vi "_Remote RT Copy.vi"(6 "Error In":errorcluster, 7 "Copy software only":bool, 8 "Image Destination":T1, 9 "Image Source":T1) -> (0 "Error Out":errorcluster, 3 "Messages":string)   [LabVIEW 2018]
uses:
  Type/_RT Command.ctl
  Type/_RT Instrument State.ctl
  Configuration/_Global Configuration.vi
  <vilib>/nisyscfg/Create System Image (Folder).vi
  <vilib>/nisyscfg/Set System Image (Folder).vi
  <vilib>/nisyscfg/Close (System).vi
  <vilib>/nisyscfg/nisyscfg.lvlib
panel:
  out "IP Address:":string
  out "Current Task":string
  # "Please wait up to a few minutes while copying firmware"
  # "(This dialog will automatically close when update is finished)"
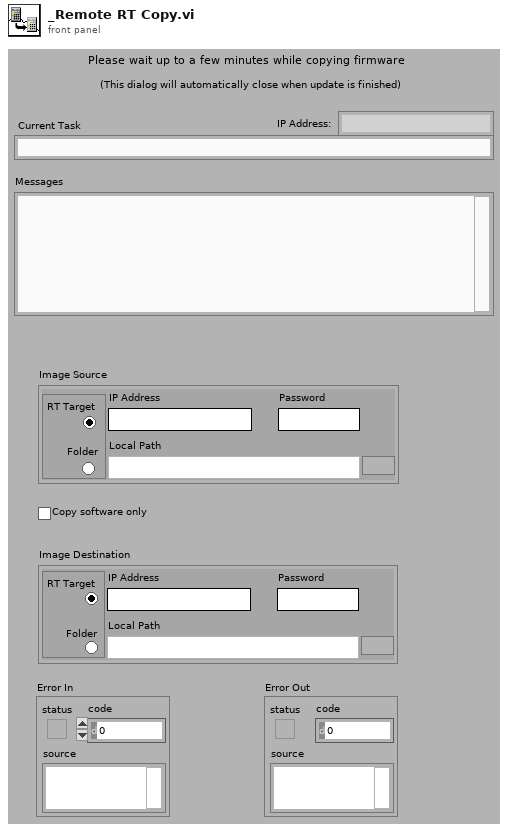
[diagram p1: front panel]
types:
  T1 = cluster{"IP Address":string, "Password ":string, "Local Path":path, "Radio Buttons":enum32{"RT Target", "Folder"}}
  T2 = typedef "_RT Command.ctl" = enum16{"xml Start Run", "xml Start Actual Run", "xml Stop Run", "xml Runtime Update", "xml Get Status", "xml Get Table", "xml Set Table", "xml Get Configuration", "xml System Status", "xml Set LC Input Logic", "xml Get Data", "xml Get Info", "Start", "StartActualRun", "Stop", "Runtime Update", "Get Data", "Get Info", "Get Status", "Get Param", "Get Config", "Get Table", "Read ADC", "Set Oscillator", "Update Config", "Update Table", "Set All Pol", "Set Pol and DC", "Set Max Mass", "Toggle RP", "Toggle EL", "Set PIC", "Initialize Turbo", "Send Turbo Comm", "Close Turbo", "P1", "P2", "P3", "Send Serial", "Set LC Out", "Get LC In", "Read VAC", "Test Table", "Toggle Power", "Get Startup", "Set Startup", "Get ADC Table", "Set ADC Table", "Get Brief Status", "Get Detail Status", "Auxiliary Update", "Set CC Logics", "Set CC Input Logics", "Ignore Error", "invalid"}
  T3 = enum16{"Use Dialog", "Temporary File", "My Tables"}
  T4 = typedef "_RT Instrument State.ctl" = enum16{"Initializing", "Mass Spectrometer is Off", "Starting Up", "Turning Power Off", "Going to Standby", "Roughing Pump Ready", "Turning Turbo Off", "Turbo Startup", "Turbopump Ready", "Checking Vacuum", "Going to Ready", "Ready", "Running", "Source Standby", "Lost Communication", "Shutting Down", "Fault", "24V Standby", "Go to 24V Standby", "Turbopump Ready-Waiting"}
  T5 = cluster{"Model":string, "MAC Address":string, "Hostname":string}
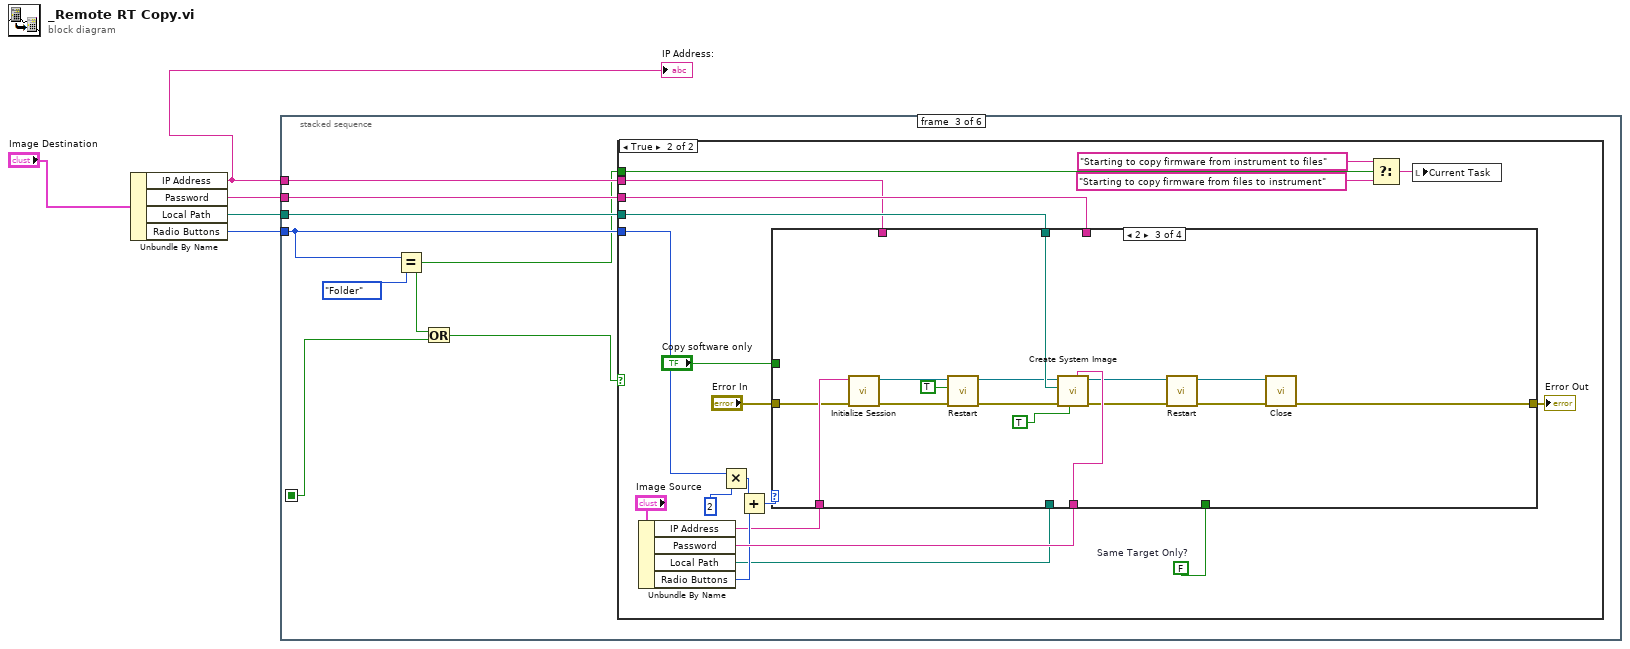
[diagram p0: block diagram]
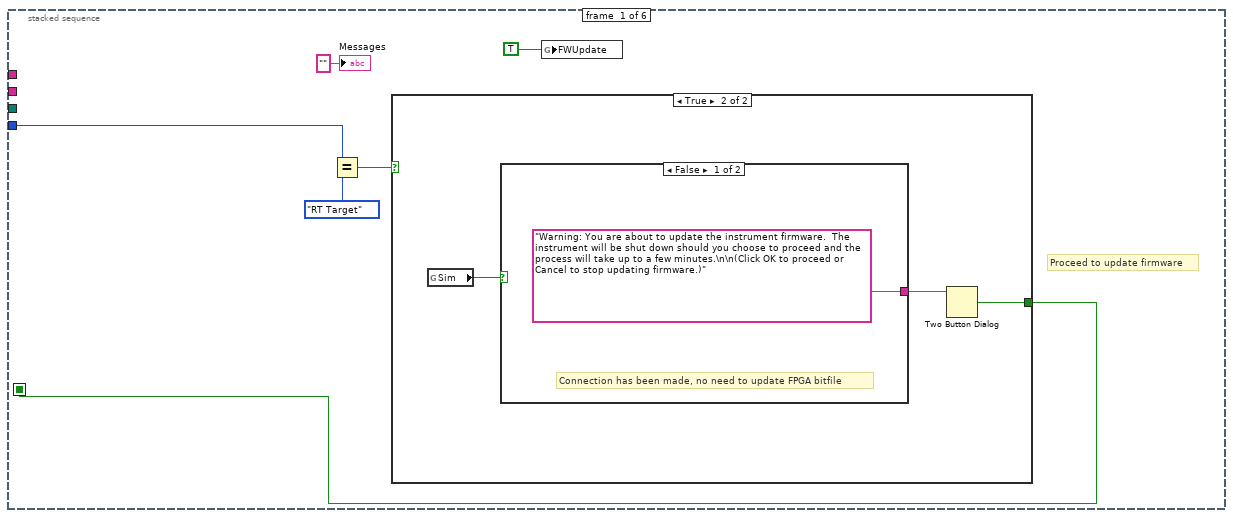
[diagram p2: hidden frame]
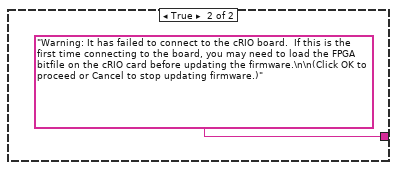
[diagram p4: hidden frame]
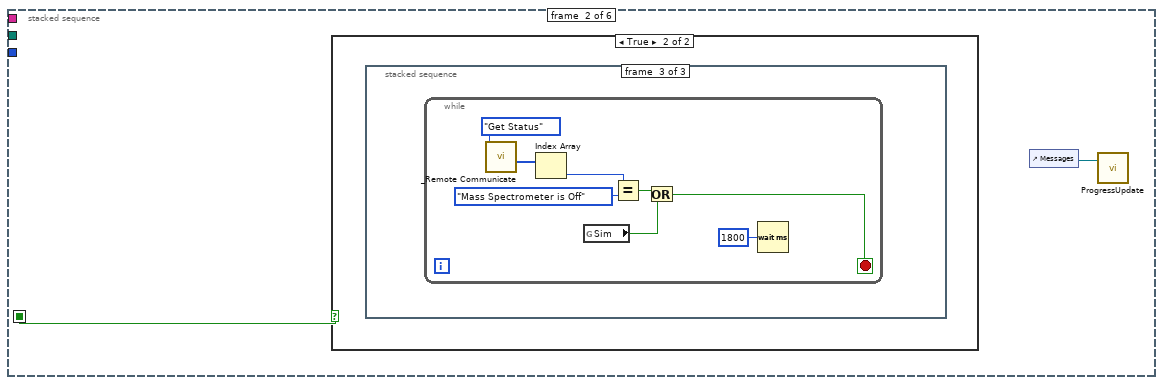
[diagram p5: hidden frame]
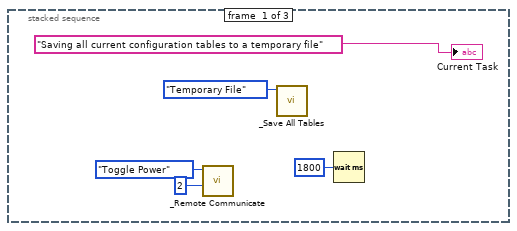
[diagram p7: hidden frame]
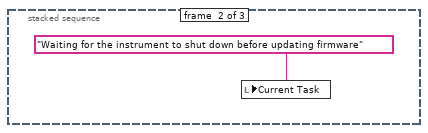
[diagram p8: hidden frame]
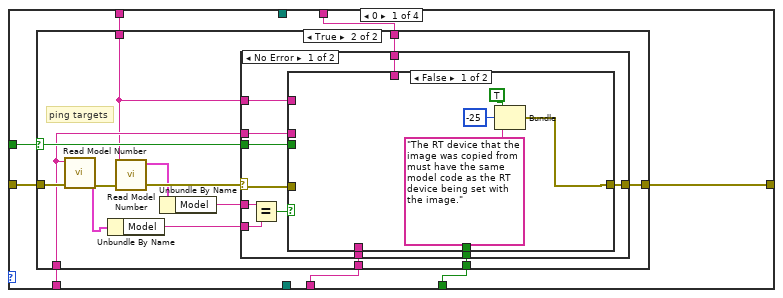
[diagram p10: hidden frame]
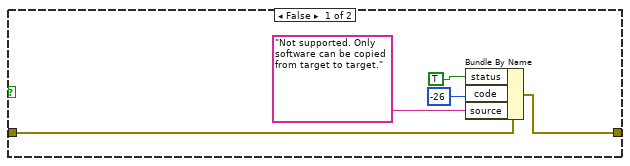
[diagram p11: hidden frame]
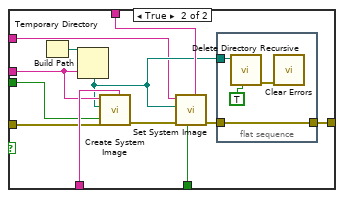
[diagram p12: hidden frame]
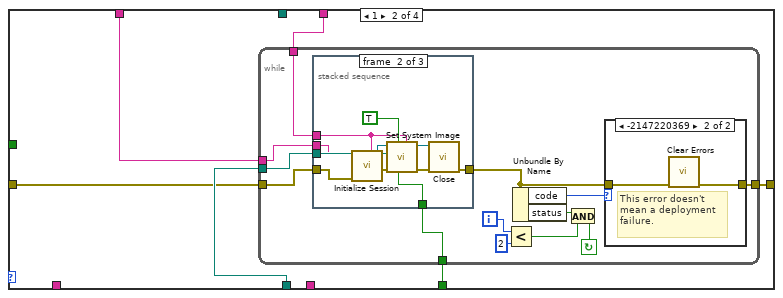
[diagram p14: hidden frame]
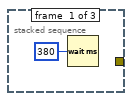
[diagram p16: hidden frame]
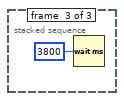
[diagram p17: hidden frame]
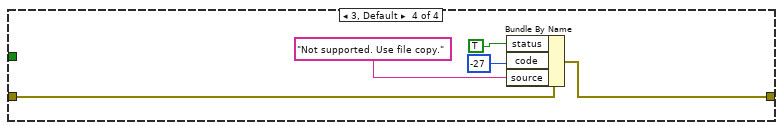
[diagram p18: hidden frame]
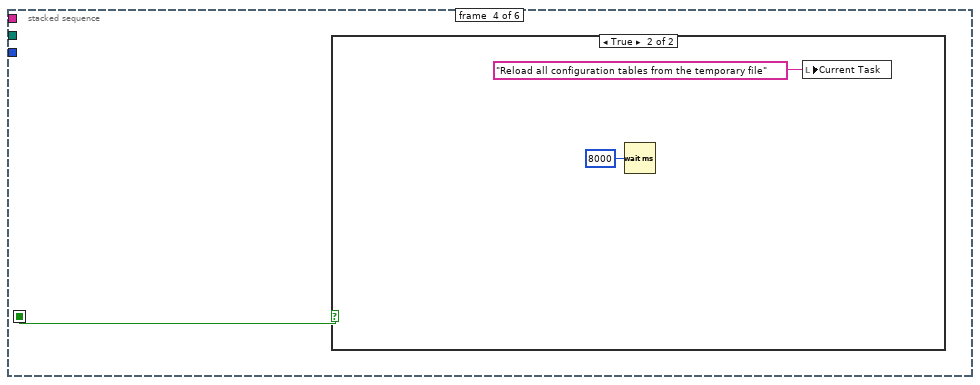
[diagram p19: hidden frame]
diagram:
  n1 = Unbundle By Name("Image Destination") -> ("IP Address"=w1:string, "Password"=w4:string, "Local Path"=w3:path, "Radio Buttons"=w2:enum32{"RT Target", "Folder"})
  "IP Address:" <- w1
  n2 = stacked-sequence {
    seq-local: [w8 _ _ _ _ _] -> [_ w19 w35 w176 w180 _]
    tunnel: w2 -> [w10 _ w37 _ _ _]
    tunnel: w4 -> [_ _ w41 _ _ _]
    tunnel: w3 -> [_ _ w40 _ _ _]
    tunnel: w1 -> [_ _ w39 _ w179 _]
    frame #0 {
      # "Proceed to update firmware"
      n3 = Equal?(x=w10, y=enum32{"RT Target", "Folder"}."RT Target") -> (x = y?=w9:bool)
      n4 = case shown="True" w9 {
        selector: w9 -> [w12 _]
        tunnel: [w12 w15] -> w8
        frame False {
        }
        frame True {
          n5 = global read "_Global Configuration.vi" "Sim"() -> (w13:bool)
          n6 = case shown="False" w13 {
            tunnel: ["Warning: You are about to update the instrument firmware.  The instrument will be shut down should you choose to proceed and the process will take up to a few minutes.\n\n(Click OK to proceed or Cancel to stop updating firmware.)" "Warning: It has failed to connect to the cRIO board.  If this is the first time connecting to the board, you may need to load the FPGA bitfile on the cRIO card before updating the firmware.\n\n(Click OK to proceed or Cancel to stop updating firmware.)"] -> w14
            frame False {
              # "Connection has been made, no need to update FPGA bitfile"
            }
            frame True {
            }
          }
          n7 = Two Button Dialog(message=w14) -> (T button?=w15:bool)  [unwired: 2 out]
        }
      }
      n8 = global write "_Global Configuration.vi" "FWUpdate"(TRUE ("Update")) -> ()
      "Messages" <- "" ("Messages")
    }
    frame #1 {
      n9 = case shown="True" w19 {
        frame False {
        }
        frame True {
          n10 = stacked-sequence {
            frame #0 {
              n11 = call "_Remote Communicate.vi"("DC Param"=u16 2, "Command"=_RT_Command."Toggle Power") -> ()  [unwired: 4 in, 4 out]
              n12 = call "_Save All Tables.vi"("SaveOption (Temporary File)"=T3."Temporary File" ("Use temporary file (F)")) -> ()  [unwired: 2 in, 5 out]
              n13 = Wait (ms)(milliseconds to wait=u32 1800) -> ()  [unwired: 1 out]
              "Current Task" <- "Saving all current configuration tables to a temporary file"
            }
            frame #1 {
              n14 = local write "Current Task"("Waiting for the instrument to shut down before updating firmware") -> ()
            }
            frame #2 {
              n15 = while {
                stop <- w27 stop-if-true
                n16 = call "_Remote Communicate.vi"("Command"=_RT_Command."Get Status") -> ("Data Array"=w32:i32[])  [unwired: 5 in, 3 out]
                n17 = Index Array(array=w32) -> (element=w31:i32)  [unwired: 1 in]
                n18 = global read "_Global Configuration.vi" "Sim"() -> (w28:bool)
                n19 = Equal?(x=w31, y=_RT_Instrument_State."Mass Spectrometer is Off" ("InstrState")) -> (x = y?=w29:bool)
                n20 = Or(x=w29, y=w28) -> (x .or. y?=w27:bool)
                n21 = Wait (ms)(milliseconds to wait=u32 1800) -> ()  [unwired: 1 out]
              }
            }
          }
        }
      }
      n22 = control-ref of="Messages"() -> (w18:refnum<vi>)
      n23 = call <userlib>:"ProgressUpdate.vi"("Progress ref"=w18) -> ()  [unwired: 1 in, 1 out]
    }
    frame #2 {
      n24 = Equal?(x=w37, y=enum32{"RT Target", "Folder"}."Folder") -> (x = y?=w34:bool)
      n25 = Or(x=w34, y=w35) -> (x .or. y?=w36:bool)
      n26 = case shown="True" w36 {
        tunnel: w37 -> [_ w58]
        tunnel: w41 -> [_ w56]
        tunnel: w40 -> [_ w51]
        tunnel: w39 -> [_ w47]
        tunnel: w34 -> [_ w42]
        frame False {
        }
        frame True {
          w46 = FALSE  # Same Target Only?
          n27 = Unbundle By Name("Image Source") -> ("IP Address"=w48:string, "Password"=w55:string, "Local Path"=w52:path, "Radio Buttons"=w53:enum32{"RT Target", "Folder"})
          n28 = Multiply(x=w58, y=2) -> (x*y=w54:u32)
          n29 = Add(x=w54, y=w53) -> (x+y=w60:u32)
          n30 = case shown="2" w60 {
            tunnel: w47 -> [w68 w126 _ _]
            tunnel: w56 -> [w69 w122 _ _]
            tunnel: w48 -> [w66 _ w167 _]
            tunnel: w55 -> [w67 _ w165 _]
            tunnel: "Copy software only" -> [w63 _ _ _]
            tunnel: w52 -> [_ w125 _ _]
            tunnel: w51 -> [_ _ w170 _]
            tunnel: "Error In" -> [w64 w123 w166 w172]
            tunnel: [w65 w124 w168 w171] -> w49
            tunnel: w46 -> [w62 w121 _ _]
            frame 0 {
              n31 = case shown="True" w63 {
                selector: w63 -> [_ w87]
                tunnel: w69 -> [_ w86]
                tunnel: w68 -> [_ w81]
                tunnel: w67 -> [_ w88]
                tunnel: w66 -> [_ w82]
                tunnel: [w71 w85] -> w65
                tunnel: w64 -> [w72 w83]
                tunnel: w62 -> [_ w79]
                frame False {
                  n32 = Bundle By Name(cluster=w72, "status"=TRUE, "code"=-26, "source"="Not supported. Only software can be copied from target to target.") -> (w71:errorcluster)
                }
                frame True {
                  # "ping targets"
                  n33 = call "Read Model Number.vi"("error in (no error)"=w83, "String"=w82) -> ("error out"=w84:errorcluster, "Target Info"=w76:T5)  [unwired: 8 in]
                  n34 = Unbundle By Name(w76) -> ("Model"=w77:string)
                  n35 = call "Read Model Number.vi"("error in (no error)"=w84, "String"=w81) -> ("error out"=w80:errorcluster, "Target Info"=w75:T5)  [unwired: 8 in]
                  n36 = Unbundle By Name(w75) -> ("Model"=w78:string)
                  n37 = case shown="No Error" w80 {
                    selector: w80 -> [w95 w120]
                    tunnel: w88 -> [w99 _]
                    tunnel: w87 -> [w98 _]
                    tunnel: w86 -> [w92 _]
                    tunnel: [w97 w120] -> w85
                    tunnel: w82 -> [w94 _]
                    tunnel: w81 -> [w96 _]
                    tunnel: w79 -> [w93 _]
                    tunnel: w78 -> [w89 _]
                    tunnel: w77 -> [w91 _]
                    frame No Error {
                      n38 = Equal?(x=w89, y=w91) -> (x = y?=w90:bool)
                      n39 = case shown="False" w90 {
                        tunnel: w99 -> [_ w114]
                        tunnel: w98 -> [_ w113]
                        tunnel: [w100 w110] -> w97
                        tunnel: w96 -> [_ w104]
                        tunnel: w95 -> [_ w109]
                        tunnel: w94 -> [_ w106]
                        tunnel: w93 -> [_ w108]
                        tunnel: w92 -> [_ w107]
                        frame False {
                          n40 = Bundle("status"=TRUE, "code"=-25, "source"="The RT device that the image was copied from must have the same model code as the RT device being set with the image.") -> (w100:errorcluster)  [unwired: 1 out]
                        }
                        frame True {
                          n41 = Temporary Directory() -> (w115:path)
                          n42 = Build Path(base path=w115, name or relative path=w106) -> (appended path=w105:path)
                          n43 = call-poly <vilib>:"Create System Image.vi"("Encryption Passphrase"=w114, "Overwrite (F)"=w113, "error in (no error)"=w109, "Destination Folder"=w105, "Session in"=w106) -> ("error out"=w112:errorcluster)  [unwired: 4 in, 2 out]
                          n44 = call-poly <vilib>:"Set System Image.vi"("Encryption Passphrase"=w107, "Original System Only (F)"=w108, "error in (no error)"=w112, "Source Folder"=w105, "Session in"=w104) -> ("error out"=w111:errorcluster)  [unwired: 5 in, 1 out]
                          n45 = flat-sequence {
                            tunnel: w111 -> [w119]
                            tunnel: [w119] -> w110
                            tunnel: w105 -> [w117]
                            frame #0 {
                              n46 = call <vilib>:"Delete Directory Recursive.vi"("keep deleting on error? (F)"=TRUE, "Folder to Delete"=w117) -> ("error out"=w116:errorcluster)  [unwired: 1 in, 8 out]
                              n47 = call <vilib>:"Clear Errors.vi"("error in (no error)"=w116) -> ()  [unwired: 1 in, 6 out]
                            }
                          }
                        }
                      }
                    }
                    frame Error {
                    }
                  }
                }
              }
            }
            frame 1 {
              n48 = while {
                tunnel: w126 -> [w139]
                tunnel: w125 -> [w138]
                tunnel: [w128] -> w124
                tunnel: w123 -> [w137]
                tunnel: w122 -> [w136]
                tunnel: w121 -> [w135]
                i -> [w132]
                stop <- w134 continue-if-true
                n49 = stacked-sequence {
                  tunnel: w139 -> [_ w145 _]
                  tunnel: w138 -> [_ w154 _]
                  tunnel: w137 -> [_ w148 _]
                  tunnel: w136 -> [_ w146 _]
                  tunnel: w135 -> [_ w153 _]
                  tunnel: [_ w149 _] -> w129
                  frame #0 {
                    n50 = Wait (ms)(milliseconds to wait=u32 380) -> ()  [unwired: 1 out]
                  }
                  frame #1 {
                    n51 = call <vilib>:"Initialize Session.vi"("Password"=w146, "error in (no error)"=w148, "Target (localhost)"=w145) -> ("error out"=w147:errorcluster, "Session out"=w144:refnum<k21>)  [unwired: 7 in]
                    n52 = call-poly <vilib>:"Set System Image.vi"("Encryption Passphrase"=w146, "Original System Only (F)"=w153, "Restart Automatically (T)"=TRUE, "error in (no error)"=w147, "Source Folder"=w154, "Session in"=w144) -> ("error out"=w150:errorcluster, "Session out"=w151:refnum<k21>)  [unwired: 4 in]
                    n53 = call-poly <vilib>:"Close.vi"("error in (no error)"=w150, "Session in"=w151) -> ("error out"=w149:errorcluster)  [unwired: 9 in]
                  }
                  frame #2 {
                    n54 = Wait (ms)(milliseconds to wait=u32 3800) -> ()  [unwired: 1 out]
                  }
                }
                n55 = Less?(x=w132, y=2) -> (x < y?=w130:bool)
                n56 = Unbundle By Name(w129) -> ("code"=w127:i32, "status"=w133:bool)
                n57 = And(x=w133, y=w130) -> (x .and. y?=w134:bool)
                n58 = case shown="-2147220369" w127 {
                  tunnel: w129 -> [w140 w142]
                  tunnel: [w140 w141] -> w128
                  frame Default {
                  }
                  frame -2147220369 {
                    # "This error doesn't\nmean a deployment\nfailure."
                    n59 = call <vilib>:"Clear Errors.vi"("error in (no error)"=w142) -> ("error out"=w141:errorcluster)  [unwired: 5 in, 1 out]
                  }
                }
              }
            }
            frame 2 {
              n60 = call <vilib>:"Initialize Session.vi"("error in (no error)"=w166, "Target (localhost)"=w167) -> ("error out"=w162:errorcluster, "Session out"=w164:refnum<k21>)  [unwired: 8 in]
              n61 = call <vilib>:"Restart.vi"("error in (no error)"=w162, "Install Mode (F)"=TRUE, "Session in"=w164) -> ("error out"=w161:errorcluster, "Session out"=w163:refnum<k21>)  [unwired: 6 in, 1 out]
              n62 = call-poly <vilib>:"Create System Image.vi"("Encryption Passphrase"=w165, "Overwrite (F)"=TRUE, "error in (no error)"=w161, "Destination Folder"=w170, "Session in"=w163) -> ("error out"=w158:errorcluster, "Session out"=w159:refnum<k21>)  [unwired: 4 in, 1 out]
              n63 = call <vilib>:"Restart.vi"("error in (no error)"=w158, "Session in"=w159) -> ("error out"=w157:errorcluster, "Session out"=w156:refnum<k21>)  [unwired: 7 in, 1 out]
              n64 = call-poly <vilib>:"Close.vi"("error in (no error)"=w157, "Session in"=w156) -> ("error out"=w168:errorcluster)  [unwired: 9 in]
            }
            frame 3, Default {
              n65 = Bundle By Name(cluster=w172, "status"=TRUE, "code"=-27, "source"="Not supported. Use file copy.") -> (w171:errorcluster)
            }
          }
          "Error Out" <- w49
          n66 = Select(t="Starting to copy firmware from instrument to files", s=w42, f="Starting to copy firmware from files to instrument") -> (s? t:f=w45:string)
          n67 = local write "Current Task"(w45) -> ()
        }
      }
    }
    frame #3 {
      n68 = case shown="True" w176 {
        frame False {
        }
        frame True {
          n69 = Wait (ms)(milliseconds to wait=u32 8000) -> ()  [unwired: 1 out]
          n70 = local write "Current Task"("Reload all configuration tables from the temporary file") -> ()
        }
      }
    }
    frame #4 {
      n71 = case shown="True" w180 {
        tunnel: w179 -> [_ w181]
        frame False {
        }
        frame True {
          n72 = flat-sequence {
            tunnel: w181 -> [w182]
            frame #0 {
              n73 = call "_Remote Connect.vi"("IP Address"=w182) -> ()  [unwired: 1 in, 6 out]
            }
            frame #1 {
              n74 = Wait (ms)(milliseconds to wait=u32 3000) -> ()  [unwired: 1 out]
            }
            frame #2 {
              n75 = call "_Load All Tables.vi"("Use temporary file (F)"=TRUE) -> ()  [unwired: 7 out]
            }
          }
        }
      }
    }
    frame #5 {
      n76 = global write "_Global Configuration.vi" "FWUpdate"(FALSE ("Update")) -> ()
    }
  }
